vi "SetPolarity.vi"(8 "error in (no error)":errorcluster, 11 "Laser Diode Controller in":refnum<class "KLD101.lvclass">) -> (0 "error out":errorcluster, 3 "Laser Diode Controller out":refnum<class "KLD101.lvclass">)   [LabVIEW 2016, in "Laser Diode Controller.lvlib" / "KLD101.lvclass"]
uses:
  KLD101.lvclass
  KLD101.lvclass/KLD101.ctl
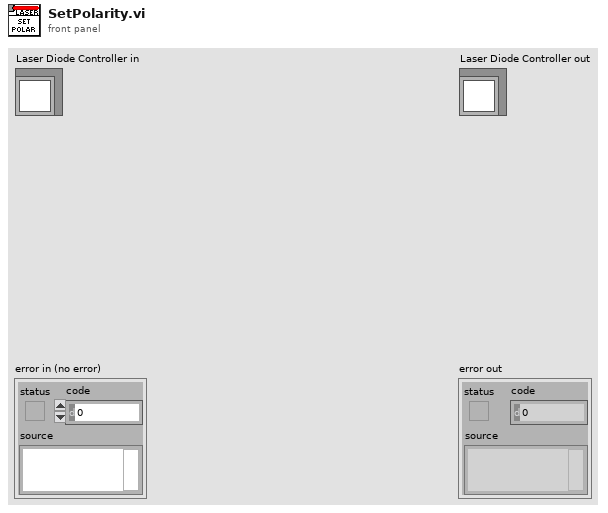
[diagram p1: front panel]
types:
  T1 = typedef "Configuration.lvlib/Config Data.lvclass/LaserPolarity.ctl" = enum16{"Anode Grounded", "Cathode Grounded"}
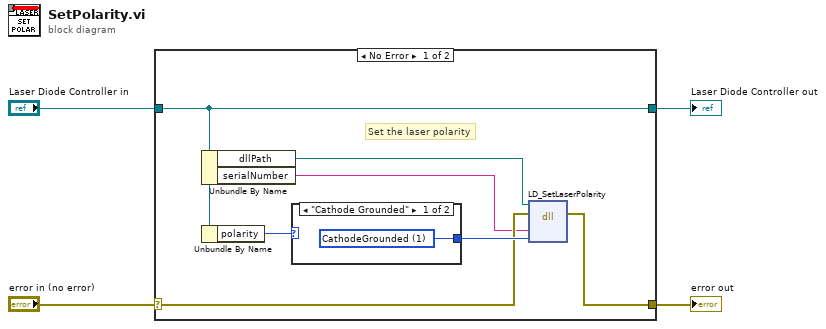
[diagram p0: block diagram]
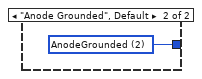
[diagram p2: hidden frame]
diagram:
  n1 = case shown="No Error" "error in (no error)" {
    selector: "error in (no error)" -> [w8 w15]
    tunnel: [w7 w15] -> w3
    tunnel: [w10 w14] -> w1
    tunnel: "Laser Diode Controller in" -> [w10 w14]
    frame No Error {
      # "Set the laser polarity"
      n2 = Unbundle By Name(w10) -> ("dllPath"=w5:path, "serialNumber"=w6:string)
      n3 = Unbundle By Name(w10) -> ("polarity"=w11:T1)
      n4 = case shown="\"Cathode Grounded\"" w11 {
        tunnel: [w12 w13] -> w9
        frame "Cathode Grounded" {
          w12 = u16 1 items=["CathodeGrounded"=1, "AnodeGrounded"=2] ("LaserPolarity")
        }
        frame "Anode Grounded", Default {
          w13 = u16 2 items=["CathodeGrounded"=1, "AnodeGrounded"=2] ("LaserPolarity")
        }
      }
      n5 = dll-call lib="C:/IDEXX Software/Collimation/data/Thorlabs.MotionControl.KCube.LaserDiode.dll" fn="LD_SetLaserPolarity"(path in=w5, error in=w8, "SerialNumber"=w6, "Polarity"=w9) -> (error out=w7:errorcluster)  [unwired: 4 in, 1 out]
    }
    frame Error {
    }
  }
  "error out" <- w3
  "Laser Diode Controller out" <- w1
